vi "1A-z-dist.vi"(5 "z ?":dbl) -> (8 "f(z)":dbl=0.3989422804014327, 10 "F(z)":dbl)   [LabVIEW 2010, in "lv_02.lvlib"]
doc: "LNCR : retourne f(z) et F(z) avec z quantile de gauss"
uses:
  <vilib>/gmath/statdist.llb/Normal CDF.vi
  <vilib>/gmath/statdist.llb/Normal PDF.vi
  lv_02.lvlib
  <vilib>/gmath/NI_Gmath.lvlib
panel:
  out "z":dbl
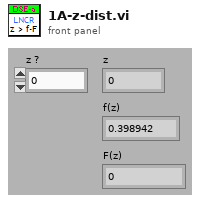
[diagram p1: front panel]
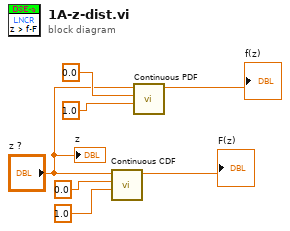
[diagram p0: block diagram]
diagram:
  n1 = call-poly <vilib>:"Continuous CDF.vi"("std"=1.0 ("mean"), "mean"=0.0 ("x"), "x"="z ?") -> ("cdf(x)"=→"F(z)":dbl)  [unwired: 7 in, 1 out]
  n2 = call-poly <vilib>:"Continuous PDF.vi"("std"=1.0 ("mean"), "mean"=0.0 ("x"), "x"="z ?") -> ("pdf(x)"=→"f(z)":dbl)  [unwired: 7 in, 1 out]
  "z" <- "z ?"
